vi "LoadObject.vi"(8 "No Error":errorcluster) -> (0 "Error Out":errorcluster, 3 "Handle [SDL_SharedObject *]":i64 format="%.0x")   [LabVIEW 2024, in "SDL3.lvlib" / "LoadSO.lvlib"]
doc: "<B>Summary</B>\nDynamically load a shared object."
uses:
  LoadSO.lvlib
  Lib/Win32/SDL3.dll
panel:
  in  "Shared Object File":string
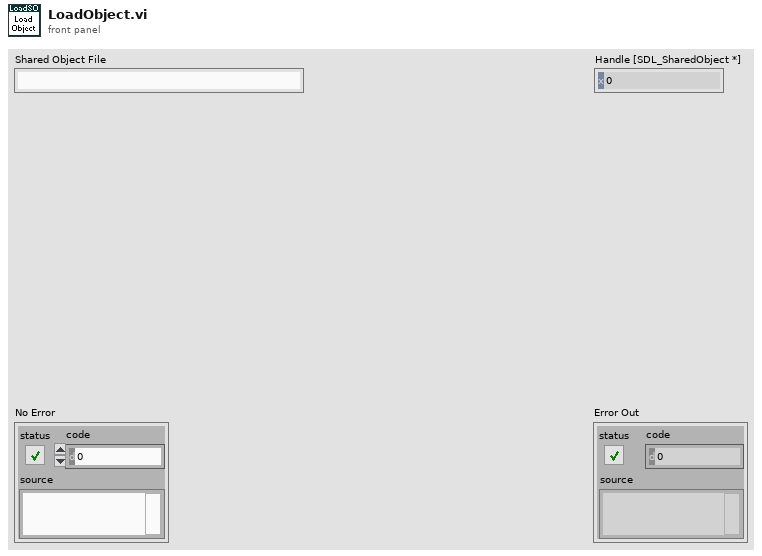
[diagram p1: front panel]
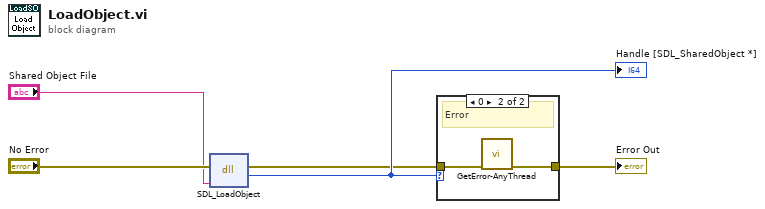
[diagram p0: block diagram]
diagram:
  n1 = dll-call lib="C:/Users/Thomas/Documents/Projects/LV-SDL3/Lib/Win32/SDL3.dll" fn="SDL_LoadObject"(error in="No Error", "sofile"="Shared Object File") -> (error out=w2:errorcluster, "return type"=w4:i64)  [unwired: 3 in, 1 out]
  "Handle [SDL_SharedObject *]" <- w4
  n2 = case shown="0" w4 {
    tunnel: w2 -> [w6 w8]
    tunnel: [w6 w7] -> w3
    frame Default {
      # "Ok"
    }
    frame 0 {
      # "Error"
      n3 = call "GetError-AnyThread.vi"("No Error"=w8) -> ("Error Out"=w7:errorcluster)  [unwired: 10 in]
    }
  }
  "Error Out" <- w3
